vi "Lab01.vi"() -> ()   [LabVIEW 2022 SP3]
panel:
  out "Array":dbl[](array[numeric])
  out "Waveform Graph":dbl[](graph)
  in  "Number of Points":i32=8 min=8 max=1000
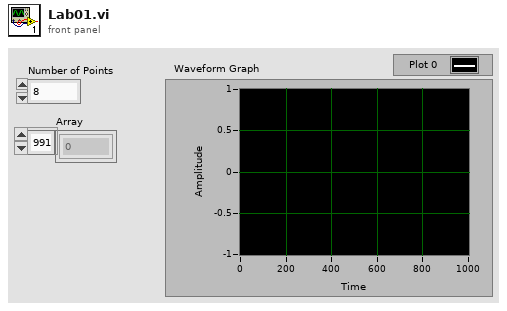
[diagram p1: front panel]
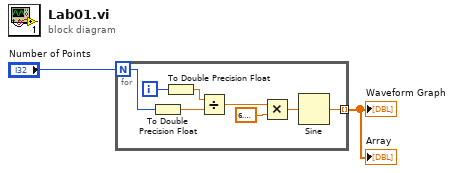
[diagram p0: block diagram]
diagram:
  n1 = for {
    N: "Number of Points" -> [w5]
    tunnel: [w6] -> w1 mode=indexing
    i -> [w10]
    n2 = To Double Precision Float(number=w5) -> (double precision float=w4:dbl)
    n3 = To Double Precision Float(number=w10) -> (double precision float=w3:dbl)
    n4 = Divide(x=w3, y=w4) -> (x/y=w8:dbl)
    n5 = Multiply(x=w8, y=6.283185307179586) -> (x*y=w7:dbl)
    n6 = Sine(x=w7) -> (sin(x)=w6:dbl)
  }
  "Waveform Graph" <- w1
  "Array" <- w1
